vi "Example2.vi"() -> ()   [LabVIEW 2020, in "LcPictureBox.lvclass"]
uses:
  LcPictureBox.lvclass
  SmoothingMode.ctl
  Pen.ctl
  <vilib>/numeric/Random Number (Range) DBL.vi
  System.Windows.Forms
panel:
  in  "PictureBox":refnum<k24>(container)
  out "TotalTime(ms)":u32
  out "error out":errorcluster
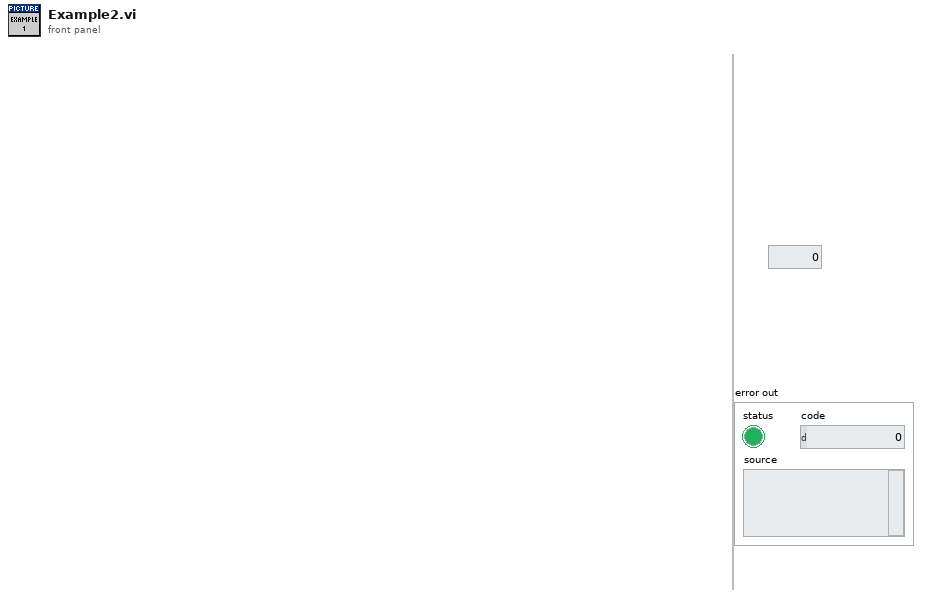
[diagram p1: front panel]
types:
  T1 = typedef "LcPictureBox.lvclass/SmoothingMode.ctl" = enum16{"None", "HighSpeed", "HighQuality", "AntiAlias"}
  T2 = typedef "LcPictureBox.lvclass/Pen.ctl" = cluster{"Width":u16, "Style":enum32{"Solid", "Dash", "Dot", "DashDot", "DashDotDot"}}
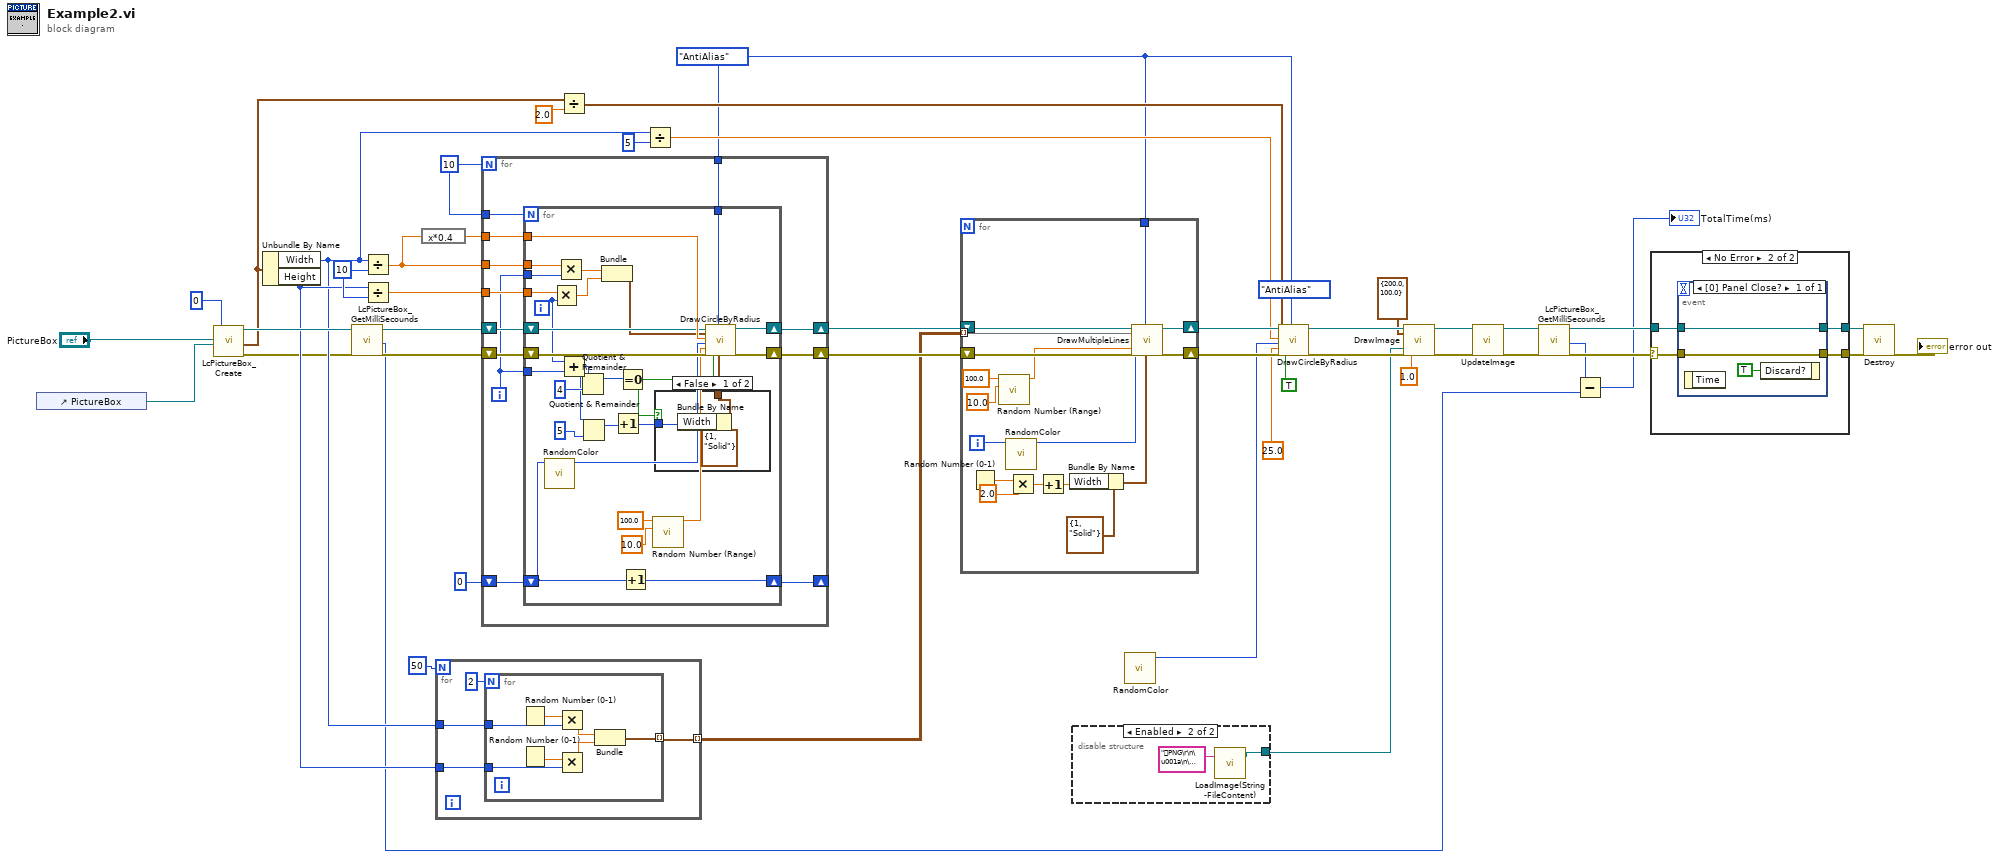
[diagram p0: block diagram]
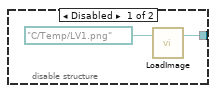
[diagram p2: hidden frame]
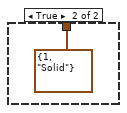
[diagram p4: hidden frame]
diagram:
  w5 = SmoothingMode."AntiAlias" ("SmoothingMode")
  (unwired) SmoothingMode."AntiAlias" ("SmoothingMode")
  w44 = 10 ("y")
  w45 = 10 ("y")
  n1 = control-ref of="PictureBox"() -> (w2:refnum<vi>)
  n2 = call "LcPictureBox_Create.vi"("PictureBox"="PictureBox", "PictureBoxActiveXReference"=w2, "CacheNumberOfPensAndColors(0)"=0 ("CacheNumberOfPensAndColors(1000)")) -> ("reference out"=w40:refnum<class "LcPictureBox.lvclass">, "ImageSizeUsed"=w30:cluster{"Width":i32, "Height":i32}, "Error Out"=w7:errorcluster)  [unwired: 14 in]
  n3 = Unbundle By Name(w30) -> ("Width"=w28:i32, "Height"=w36:i32)
  n4 = call "LcPictureBox_GetMilliSecounds.vi"("error in (no error)"=w7) -> ("msValue"=w9:u32, "error out"=w12:errorcluster)  [unwired: 17 in]
  n5 = Divide(x=w28, y=w45) -> (x/y=w42:dbl)
  n6 = Divide(x=w36, y=w45) -> (x/y=w43:dbl)
  n7 = expression code="x*0.4"(w42) -> (w41:dbl)
  n8 = for {
    N: 50 -> [_]
    tunnel: w28 -> [w48]
    tunnel: w36 -> [w47]
    tunnel: [w46] -> w34 mode=indexing
    n9 = for {
      N: 2 -> [_]
      tunnel: w48 -> [w55]
      tunnel: w47 -> [w53]
      tunnel: [w50] -> w46 mode=indexing
      n10 = Random Number (0-1)() -> (number: 0 to 1=w56:dbl)
      n11 = Random Number (0-1)() -> (number: 0 to 1=w54:dbl)
      n12 = Multiply(x=w56, y=w55) -> (x*y=w52:dbl)
      n13 = Multiply(x=w54, y=w53) -> (x*y=w51:dbl)
      n14 = Bundle(w52, w51) -> (w50:cluster{dbl, dbl})  [unwired: 1 in]
    }
  }
  n15 = for {
    N: w44 -> [_]
    tunnel: w44 -> [w68]
    tunnel: w42 -> [w67]
    tunnel: w43 -> [w66]
    tunnel: w41 -> [w65]
    shift-right: [w63] -> w38
    shift-left: w40 -> [w64]
    shift-right: [w62] -> w37
    shift-left: w12 -> [w61]
    shift-right: [w58] -> _
    shift-left: 0 ("y") -> [w59]
    tunnel: w5 -> [w57]
    i -> [w60]
    n16 = for {
      N: w68 -> [_]
      tunnel: w67 -> [w96]
      tunnel: w60 -> [w95]
      tunnel: w66 -> [w93]
      tunnel: w65 -> [w91]
      shift-right: [w89] -> w63
      shift-left: w64 -> [w90]
      shift-right: [w88] -> w62
      shift-left: w61 -> [w87]
      tunnel: w60 -> [w83]
      shift-right: [w77] -> w58
      shift-left: w59 -> [w81]
      tunnel: w57 -> [w69]
      i -> [w84]
      n17 = call "RandomColor.vi"("Index"=w81) -> ("Color"=w82:u32)  [unwired: 10 in]
      n18 = Multiply(x=w93, y=w84) -> (x*y=w92:dbl)
      n19 = Multiply(x=w96, y=w95) -> (x*y=w94:dbl)
      n20 = Add(x=w84, y=w83) -> (x+y=w73:i32)
      n21 = Quotient & Remainder(x=w73, y=4) -> (x-y*floor(x/y)=w85:i32)  [unwired: 1 out]
      n22 = Quotient & Remainder(x=w73, y=5) -> (x-y*floor(x/y)=w72:i32)  [unwired: 1 out]
      n23 = Bundle(w94, w92) -> (w70:cluster{dbl, dbl})  [unwired: 1 in]
      n24 = Increment(x=w72) -> (x+1=w71:i32)
      n25 = Equal To 0?(x=w85) -> (x = 0?=w76:bool)
      n26 = Increment(x=w81) -> (x+1=w77:i32)
      n27 = call-poly <vilib>:"Random Number (Range).vi"("lower bound (0)"=10.0, "upper bound (100)"=100.0) -> ("number"=w78:dbl)  [unwired: 9 in]
      n28 = case shown="False" w76 {
        tunnel: [w99 T2 {"Width"=1, "Style"=enum."Solid"} ("Pen(Width=1, Solid)")] -> w75
        tunnel: w71 -> [w97 _]
        frame False {
          n29 = Bundle By Name(cluster=T2 {"Width"=1, "Style"=enum."Solid"} ("Pen(Width=1, Solid)"), "Width"=w97) -> (w99:T2)
        }
        frame True {
        }
      }
      n30 = call-dynamic "DrawCircleByRadius.vi"("reference in"=w90, "Center"=w70, "Radius"=w91, "Color(Black)"=w82, "Alpha(100%)"=w78, "Error In"=w87, "Fill(False)"=w76, "SmoothingMode(AntiAlias)"=w69, "Pen(Width=1, Solid)"=w75) -> ("reference out"=w89:refnum<class "LcPictureBox.lvclass">, "Error Out"=w88:errorcluster)  [unwired: 9 in]
    }
  }
  n31 = Divide(x=w30, y=2.0 ("lower bound (0)")) -> (x/y=w26:cluster{"Width":dbl, "Height":dbl})
  n32 = Divide(x=w28, y=5) -> (x/y=w25:dbl)
  n33 = for {
    tunnel: w34 -> [w113] mode=indexing
    shift-right: [w115] -> w33
    shift-left: w38 -> [w117]
    shift-right: [w114] -> w32
    shift-left: w37 -> [w116]
    tunnel: w5 -> [w101]
    i -> [w112]
    n34 = Random Number (0-1)() -> (number: 0 to 1=w107:dbl)
    n35 = call-poly <vilib>:"Random Number (Range).vi"("lower bound (0)"=10.0, "upper bound (100)"=100.0) -> ("number"=w108:dbl)  [unwired: 9 in]
    n36 = call "RandomColor.vi"("Index"=w112) -> ("Color"=w111:u32)  [unwired: 10 in]
    n37 = Multiply(x=w107, y=2.0) -> (x*y=w105:dbl)
    n38 = Increment(x=w105) -> (x+1=w104:dbl)
    n39 = Bundle By Name(cluster=T2 {"Width"=1, "Style"=enum."Solid"} ("Pen(Width=1, Solid)"), "Width"=w104) -> (w102:T2)
    n40 = call-dynamic "DrawMultipleLines.vi"("reference in"=w117, "LineEndPoints"=w113, "Color(Black)"=w111, "Alpha(100%)"=w108, "Error In"=w116, "SmoothingMode(AntiAlias)"=w101, "Pen(Width=1, Solid)"=w102) -> ("reference out"=w115:refnum<class "LcPictureBox.lvclass">, "Error Out"=w114:errorcluster)  [unwired: 11 in]
  }
  n41 = disable-structure shown="Enabled" {
    disable-tunnel: [w118 w121] -> w1
    frame Disabled {
      n42 = call "LoadImage.vi"("ImageFile"=path "C:/Temp/LV1.png" ("Filename")) -> ("ImageOut"=w118:refnum<k24>)  [unwired: 16 in, 2 out]
    }
    frame Enabled {
      n43 = call "LoadImage(String-FileContent).vi"("ImageFileContent"="PNG\r\n\u001a\n\u0000\u0000\u0000\rIHDR\u0000\u0000\u0000ß\u0000\u0000\u0000â\b\u0003\u0000\u0000\u0000ùÃâm\u0000\u0000\u0000PLTEÿÚ\u001cÿÿÿ\u0000\u0000\u0000ÿ×\u0000ÿýôÿÙ\u0000ÿá\u001dÿÝ\u001cÿß\u001d¡\u0012n\u000eUI\tÉ¬\u0016îÌ\u001aÿã\u001dÿÚ\u0015:1\u0006¼ \u0015ÿùãÿäoÿìÿï²ÿý÷ÿÞBÿûîÿ÷Ûÿð¸ÿôÉÿöÔÿåzÿêÿéÿæÿá_ÿßKÿí©ÿòÀÿÞGÿàTÿÜ2ÿêÿäsÿùáöÓ\u001b\u0011we\rÿÝ8ÿâfl\\\f'!\u0004J?\btÙ\u0000\u0000\u0006\u0001IDATxíÝSÓL\u0010\u0007ð«á@}(\u0014ÆÒP\u0014\u0015Ô÷ÿâ\\[´K²¹ìÞþ\u0018¿ÿ1Óéä3´ý6Éºí¸Ý\u001föªéòqu}~~}u²¼<æ:&Ììø¦w÷¾ÜÆûâä#ßqaå¯ªi®²øª^øä\u0015.\u0012_,÷X\u000fot¶¾(ÏpësÏ_»ÂÅ\u0019ï1ÉÆ÷Å·òÐ_2\u001fez6¾NÞZøù8S³öMû|A8å>Ô¤¬}\u001dï¾]ágîMHðUý¿¾°Ô'\f¾9Ð\u0017§Ü\u0007<0Á\u0007æÕÿÒx7ã>äA©}\u0017\u0003|AxwÃ}Ð\u0003â@zµï\nòéùLøPq\u001f80nÐÛoGx®Cè&{mÿZ÷\bëOÜ\u0007\u000fH²/\bW\u0017Üß\u0011¾ ¼ºç\u0006ôd/\b\u001fe×4#}Ax\"Y8Ú'¼¦Að\u0011.Uâ\u0013\\Ó ùÄÖ4h¾0\u0000\u000b\u0014\"úD\u0016Q¨>5\r²O\u0010Ý'¬\"ðªiH|µÐ\t\u0011\u0012ùÄ\u0014QT>)5\rOFMCéPÓÐúðµ¦¡öq\u0017Qô>Þ\"*...") -> ("ImageOut"=w121:refnum<k24>)  [unwired: 16 in, 2 out]
    }
  }
  n44 = call "RandomColor.vi"() -> ("Color"=w23:u32)  [unwired: 11 in]
  n45 = call-dynamic "DrawCircleByRadius.vi"("reference in"=w33, "Center"=w26, "Radius"=w25, "Color(Black)"=w23, "Alpha(100%)"=25.0, "Error In"=w32, "Fill(False)"=TRUE, "SmoothingMode(AntiAlias)"=w5) -> ("reference out"=w20:refnum<class "LcPictureBox.lvclass">, "Error Out"=w22:errorcluster)  [unwired: 10 in]
  n46 = call-dynamic "DrawImage.vi"("reference in"=w20, "UpperLeftCorner(0,0)"=cluster{"x":sgl, "y":sgl} {"x"=200.0, "y"=100.0} ("UpperLeftCorner"), "Image"=w1, "Error In"=w22, "ScaleFactor(1)"=1.0) -> ("reference out"=w19:refnum<class "LcPictureBox.lvclass">, "Error Out"=w21:errorcluster)  [unwired: 13 in]
  n47 = call-dynamic "UpdateImage.vi"("reference in"=w19, "Error In"=w21) -> ("reference out"=w14:refnum<class "LcPictureBox.lvclass">, "Error Out"=w16:errorcluster)  [unwired: 14 in, 2 out]
  n48 = call "LcPictureBox_GetMilliSecounds.vi"("error in (no error)"=w16) -> ("msValue"=w10:u32, "error out"=w11:errorcluster)  [unwired: 17 in]
  n49 = Subtract(x=w10, y=w9) -> (x-y=→"TotalTime(ms)":u32)
  n50 = case shown="No Error" w11 {
    selector: w11 -> [w123 w124]
    tunnel: [w123 w127] -> w15
    tunnel: w14 -> [w122 w126]
    tunnel: [w122 w125] -> w13
    frame Error {
    }
    frame No Error {
      n51 = event shown="[0] Panel Close?" {
        selector: _ -> [_]
        dyn-events: _ -> [_]
        timeout: _ -> [_]
        tunnel: w124 -> [w129]
        tunnel: [w129] -> w127
        tunnel: w126 -> [w128]
        tunnel: [w128] -> w125
        event Panel Close? {
          n52 = event-data() -> ()  [unwired: 1 in, 1 out]
          n53 = event-data("Discard?"=TRUE) -> ()  [unwired: 1 in, 1 out]
        }
      }
    }
  }
  n54 = call-dynamic "Destroy.vi"("reference in"=w13, "Error In"=w15) -> ("Error Out"=→"error out":errorcluster)  [unwired: 16 in, 1 out]
